vi "Test Helper Loop Cannot Launch Outside Process.vi"(8 "error in (no error)":errorcluster, 11 "Helper Loop Test In":refnum<class "Helper Loop Test.lvclass">) -> (0 "error out":errorcluster, 3 "Helper Loop Test Out":refnum<class "Helper Loop Test.lvclass">)   [LabVIEW 2020, in "Helper Loop Test.lvclass"]
uses:
  Helper Loop Test.lvclass
  Mock Process/Mock Process.lvclass
  C:/Users/anton/Documents/GitHub/Triarc-Framework/source/Framework/Process/Process.lvclass
  C:/Users/anton/Documents/GitHub/Triarc-Framework/source/Framework/Base/Base.lvclass
  C:/Users/anton/Documents/GitHub/Triarc-Framework/source/Framework/Error Handler Interface/Error Handler Interface.lvclass
  C:/Users/anton/Documents/GitHub/Triarc-Framework/source/Framework/Logging/Logging.lvclass
  C:/Users/anton/Documents/GitHub/Triarc-Framework/source/Framework Test/Mock Process/Mock Process.lvclass
  C:/Users/anton/Documents/GitHub/Triarc-Framework/source/Framework/Helper Loop/Helper Loop.lvclass
  Framework/Process/Process.lvclass
  <vilib>/Asteme/LUnit/Test Case.lvclass
  C:/Program Files (x86)/National Instruments/LabVIEW 2020/vi.lib/Asteme/LUnit/Test Case.lvclass
  C:/Users/anton/Documents/GitHub/Triarc-Framework/source/Framework Test/Helper Loop Test/Helper Loop Test.lvclass
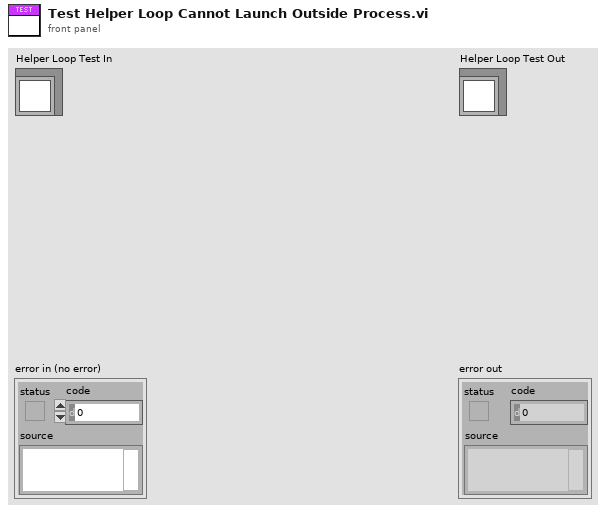
[diagram p1: front panel]
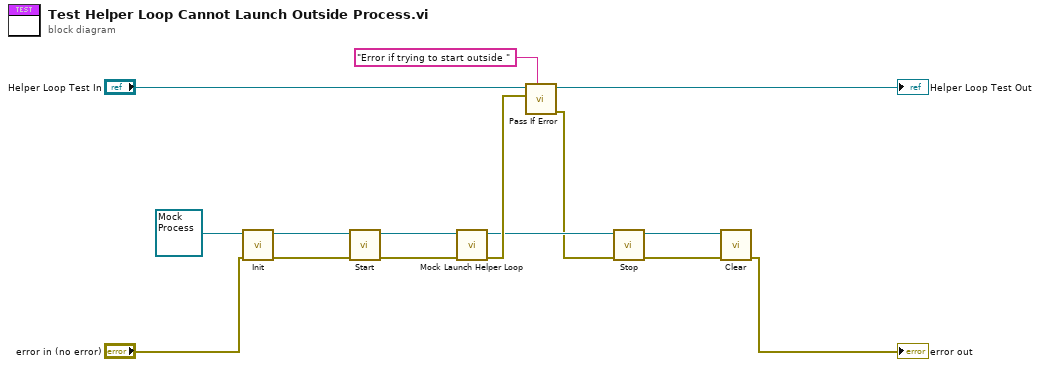
[diagram p0: block diagram]
diagram:
  n1 = call-dynamic "Init.vi"("error in (no error)"="error in (no error)", "Mock Process In"=refnum<class "Mock Process.lvclass"> refnum ("Mock Process.lvclass")) -> ("error out"=w8:errorcluster, "Mock Process Out"=w13:refnum<class "Mock Process.lvclass">)  [unwired: 8 in]
  n2 = call "Start.vi"("error in (no error)"=w8, "Process In"=w13) -> ("error out"=w7:errorcluster, "Process Out"=w12:refnum<class "Mock Process.lvclass">)  [unwired: 8 in]
  n3 = call "Mock Launch Helper Loop.vi"("error in (no error)"=w7, "Mock Process in"=w12) -> ("error out"=w10:errorcluster, "Mock Process out"=w9:refnum<class "Mock Process.lvclass">)  [unwired: 8 in]
  n4 = call <vilib>:"Pass If Error.vi"("Description"="Error if trying to start outside ", "Assert error"=w10, "Test Case In"="Helper Loop Test In") -> ("error out"=w4:errorcluster, "Test Case Out"=→"Helper Loop Test Out":refnum<class "Helper Loop Test.lvclass">)  [unwired: 7 in]
  n5 = call "Stop.vi"("error in (no error)"=w4, "Process In"=w9) -> ("error out"=w5:errorcluster, "Process Out"=w6:refnum<class "Mock Process.lvclass">)  [unwired: 7 in, 1 out]
  n6 = call-dynamic "Clear.vi"("error in (no error)"=w5, "Mock Process In"=w6) -> ("error out"=→"error out":errorcluster)  [unwired: 9 in]
